vi "record_tsv_CCP.vi"(1 "use_nfs_disk_also":bool=TRUE, 2 "use_date_folder":bool=TRUE, 3 "logging_on":bool=TRUE, 5 "file_name":string="record", 6 "error in":errorcluster, 7 "folder_name":string="subsystem", 8 "format_array":string[](array[string]), 9 "value_array":dbl[](array[numeric])=[0.0], 10 "format":string, 11 "time":timestamp) -> (0 "status":bool, 4 "error out":errorcluster)   [LabVIEW 2019]
uses:
  <vilib>/Utility/file.llb/Write Delimited Spreadsheet (string).vi
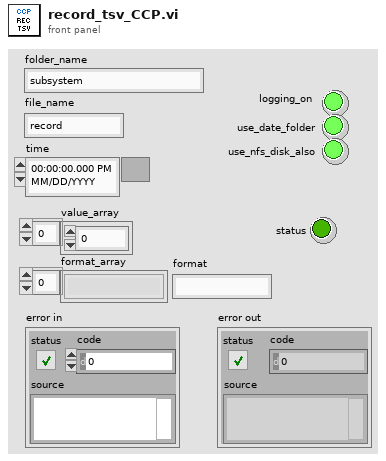
[diagram p1: front panel]
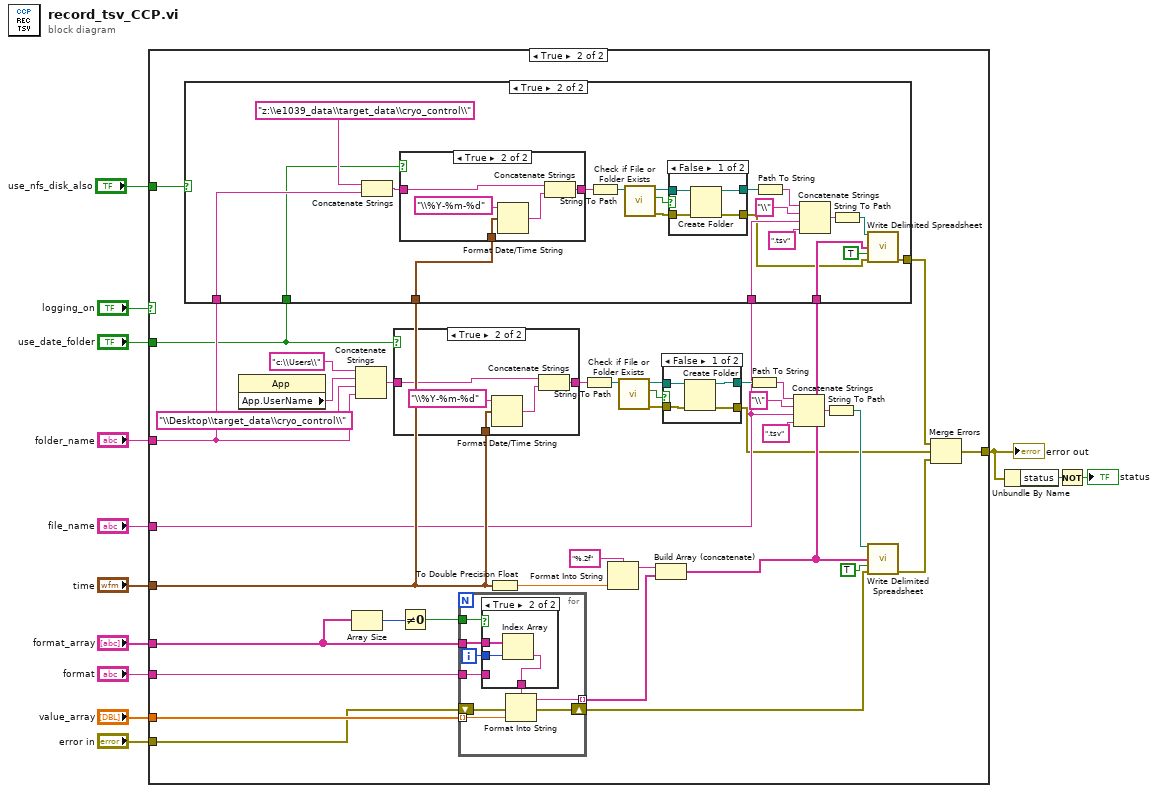
[diagram p0: block diagram]
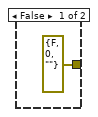
[diagram p3: hidden frame]
diagram:
  n1 = case shown="True" "logging_on" {
    tunnel: "file_name" -> [_ w24]
    tunnel: "folder_name" -> [_ w26]
    tunnel: "value_array" -> [_ w35]
    tunnel: [w14 w20] -> w4
    tunnel: "format_array" -> [_ w31]
    tunnel: "use_date_folder" -> [_ w22]
    tunnel: "time" -> [_ w25]
    tunnel: "error in" -> [w14 w28]
    tunnel: "use_nfs_disk_also" -> [_ w21]
    tunnel: "format" -> [_ w15]
    frame False {
    }
    frame True {
      n2 = property class="App"() -> ("App.UserName"=w48:string)  [unwired: 2 in, 2 out]
      n3 = Array Size(array=w31) -> (size(s)=w30:i32)
      n4 = Concatenate Strings("c:\\Users\\", w48, "\\Desktop\\target_data\\cryo_control\\", w26) -> (w33:string)
      n5 = case shown="True" w22 {
        tunnel: w33 -> [w86 w91]
        tunnel: [w86 w90] -> w32
        tunnel: w25 -> [_ w89]
        frame False {
        }
        frame True {
          n6 = Format Date/Time String(time format string (%c)="\\%Y-%m-%d", seconds (now)=w89) -> (date/time string=w87:string)  [unwired: 1 in]
          n7 = Concatenate Strings(w91, w87) -> (w90:string)
        }
      }
      n8 = Not Equal To 0?(x=w30) -> (x != 0?=w29:bool)
      n9 = for {
        tunnel: [w100] -> w34 mode=indexing
        tunnel: w35 -> [w99] mode=indexing
        tunnel: w31 -> [w96]
        tunnel: w29 -> [w98]
        shift-right: [w94] -> w27
        shift-left: w28 -> [w95]
        tunnel: w15 -> [w92]
        i -> [w93]
        n10 = case shown="True" w98 {
          tunnel: [w101 w104] -> w97
          tunnel: w96 -> [_ w103]
          tunnel: w93 -> [_ w102]
          tunnel: w92 -> [w101 _]
          frame False {
          }
          frame True {
            n11 = Index Array(array=w103, index=w102) -> (element=w104:string)
          }
        }
        n12 = Format Into String(format string=w97, error in=w95, w99) -> (resulting string=w100:string, error out=w94:errorcluster)  [unwired: 1 in]
      }
      n13 = To Double Precision Float(number=w25) -> (double precision float=w37:dbl)
      n14 = String To Path(string=w32) -> (path=w43:path)
      n15 = Format Into String(format string="%.2f", w37) -> (resulting string=w51:string)  [unwired: 2 in, 1 out]
      n16 = call <vilib>:"Check if File or Folder Exists.vi"("path"=w43) -> ("error out"=w19:errorcluster, "file or folder exists?"=w42:bool, "dup path"=w40:path)  [unwired: 8 in]
      n17 = Build Array (concatenate)(w51, w34) -> (w23:string[])
      n18 = case shown="True" w21 {
        tunnel: w26 -> [_ w62]
        tunnel: w25 -> [_ w61]
        tunnel: w24 -> [_ w60]
        tunnel: w23 -> [_ w57]
        tunnel: w22 -> [_ w56]
        tunnel: [errorcluster {"status"=FALSE, "code"=0, "source"=""} ("error out") w53] -> w16
        frame False {
        }
        frame True {
          n19 = Concatenate Strings("z:\\e1039_data\\target_data\\cryo_control\\", w62) -> (w64:string)
          n20 = case shown="True" w56 {
            tunnel: w64 -> [w74 w79]
            tunnel: [w74 w78] -> w63
            tunnel: w61 -> [_ w77]
            frame False {
            }
            frame True {
              n21 = Format Date/Time String(time format string (%c)="\\%Y-%m-%d", seconds (now)=w77) -> (date/time string=w75:string)  [unwired: 1 in]
              n22 = Concatenate Strings(w79, w75) -> (w78:string)
            }
          }
          n23 = String To Path(string=w63) -> (path=w69:path)
          n24 = call <vilib>:"Check if File or Folder Exists.vi"("path"=w69) -> ("error out"=w55:errorcluster, "file or folder exists?"=w68:bool, "dup path"=w66:path)  [unwired: 8 in]
          n25 = case shown="False" w68 {
            tunnel: w66 -> [w83 w85]
            tunnel: [w82 w85] -> w67
            tunnel: w55 -> [w81 w84]
            tunnel: [w80 w84] -> w54
            frame False {
              n26 = Create Folder(path (use dialog)=w83, error in=w81) -> (created path=w82:path, error out=w80:errorcluster)  [unwired: 1 in, 1 out]
            }
            frame True {
            }
          }
          n27 = Path To String(path=w67) -> (string=w65:string)
          n28 = Concatenate Strings(w65, "\\", w60, ".tsv" ("string")) -> (w70:string)
          n29 = String To Path(string=w70) -> (path=w59:path)
          n30 = call-poly <vilib>:"Write Delimited Spreadsheet.vi"("file path (dialog if empty)"=w59, "1D data"=w57, "append to file? (new file:F)"=TRUE, "error in (no error)"=w54) -> ("error out"=w53:errorcluster)  [unwired: 10 in, 1 out]
        }
      }
      n31 = case shown="False" w42 {
        tunnel: w40 -> [w108 w110]
        tunnel: [w107 w110] -> w41
        tunnel: w19 -> [w106 w109]
        tunnel: [w105 w109] -> w18
        frame False {
          n32 = Create Folder(path (use dialog)=w108, error in=w106) -> (created path=w107:path, error out=w105:errorcluster)  [unwired: 1 in, 1 out]
        }
        frame True {
        }
      }
      n33 = Path To String(path=w41) -> (string=w39:string)
      n34 = Concatenate Strings(w39, "\\", w24, ".tsv" ("string")) -> (w44:string)
      n35 = String To Path(string=w44) -> (path=w38:path)
      n36 = call-poly <vilib>:"Write Delimited Spreadsheet.vi"("file path (dialog if empty)"=w38, "1D data"=w23, "append to file? (new file:F)"=TRUE, "error in (no error)"=w27) -> ("error out"=w17:errorcluster)  [unwired: 10 in, 1 out]
      n37 = Merge Errors(w16, w18, w17) -> (w20:errorcluster)
    }
  }
  "error out" <- w4
  n38 = Unbundle By Name(w4) -> ("status"=w3:bool)
  n39 = Not(x=w3) -> (.not. x?=→"status":bool)
